vi "Read configuration.vi"(8 "error in":errorcluster, 11 "Scaling editor node in":refnum<class "Scaling editor node.lvclass">) -> (0 "error out":errorcluster, 2 "configuration":refnum<class "NISE_CEF_serializable configuration.lvclass">, 3 "Scaling editor node out":refnum<class "Scaling editor node.lvclass">)   [LabVIEW 2013, in "Scaling editor node.lvclass"]
uses:
  Scaling editor node.lvclass
  <vilib>/NI/Configuration Framework/serializable configuration/NISE_CEF_serializable configuration.lvclass
  Scaling editor node.lvclass/Scaling editor node.ctl
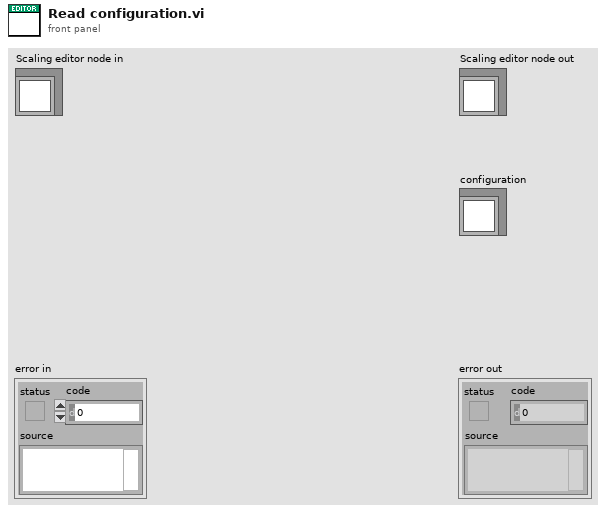
[diagram p1: front panel]
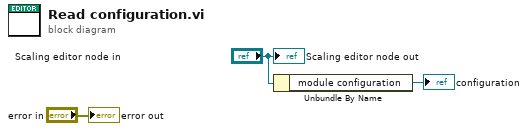
[diagram p0: block diagram]
diagram:
  n1 = Unbundle By Name("Scaling editor node in") -> ("module configuration"=→"configuration":refnum<class "Scaling configuration.lvclass">)
  "error out" <- "error in"
  "Scaling editor node out" <- "Scaling editor node in"
